vi "2D array remove NaN.vi"(1 "Data array":bool, 2 "2D array IN":dbl[][](array[numeric])=[[1.0, nan, 3.0], [1.0, 3.0, 4.0], [4.0, 5.0, nan], [5.0, 7.0, 6.0], [0.0, 0.0, 7.0]], 3 "delete Nan":bool) -> (0 "2D array cleaned":dbl[][](array[numeric])=[[1.0, 3.0, 4.0], [5.0, 7.0, 6.0], [0.0, 0.0, 7.0]])   [LabVIEW 2021]
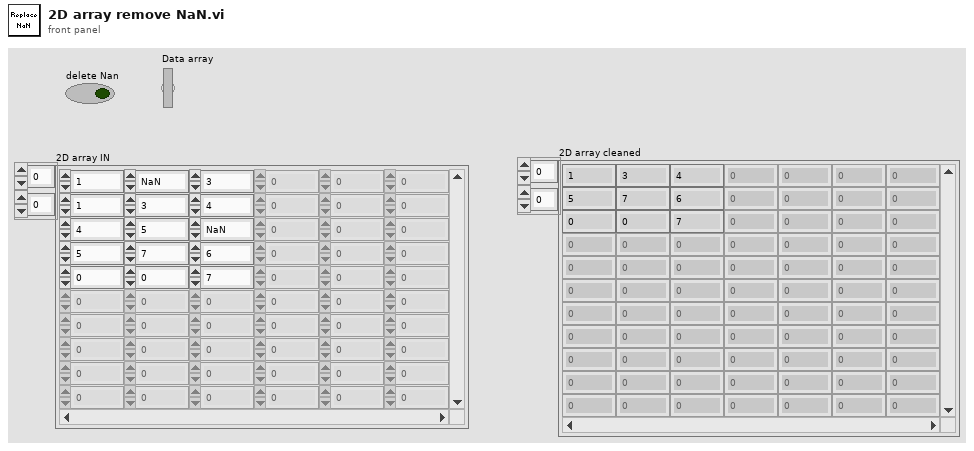
[diagram p1: front panel]
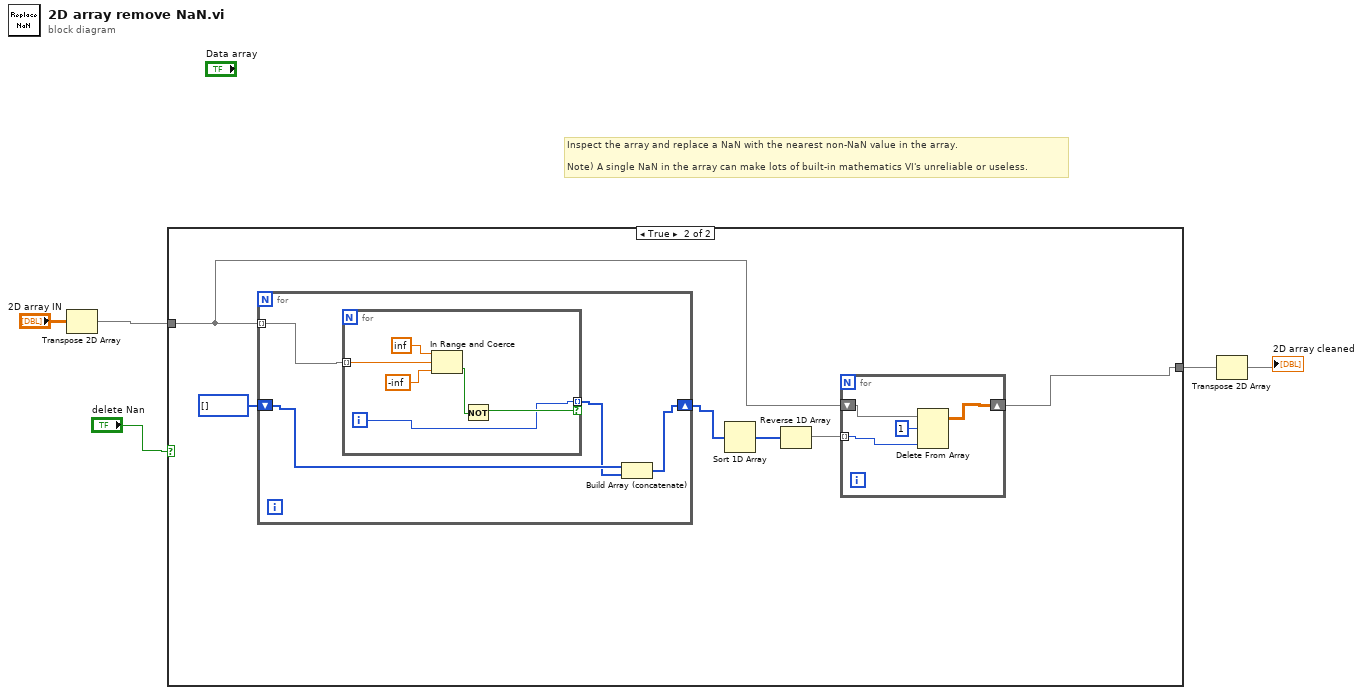
[diagram p0: block diagram]
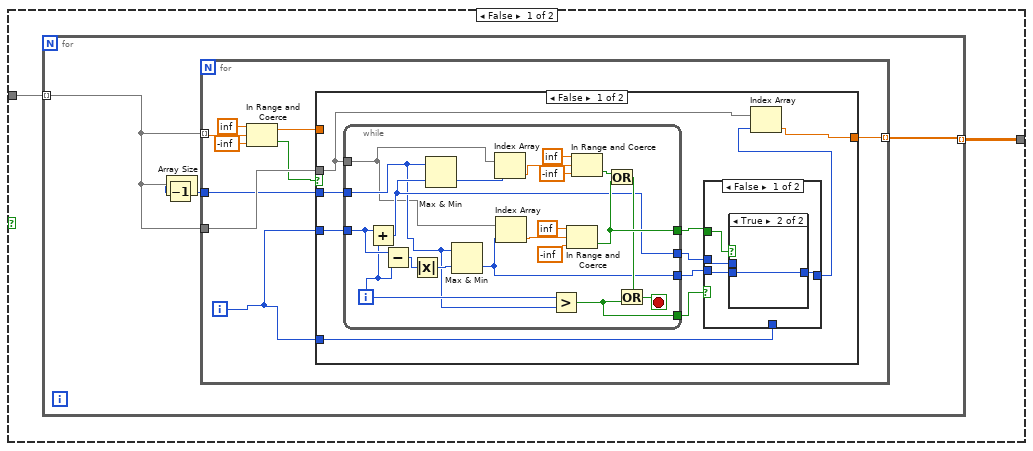
[diagram p2: hidden frame]
diagram:
  # "Inspect the array and replace a NaN with the nearest non-NaN value in the array.\n\nNote) A single NaN in the array can make lots of built-in mathematics VI's unreliable or useless."
  n1 = Transpose 2D Array(2D array="2D array IN") -> (transposed array=w3:dbl[][])
  n2 = case shown="True" "delete Nan" {
    tunnel: [w7 w59] -> w4
    tunnel: w3 -> [w6 w63]
    frame False {
      n3 = for {
        tunnel: w6 -> [w11] mode=indexing
        tunnel: [w10] -> w7 mode=indexing
        n4 = Array Size(array=w11) -> (size(s)=w9:i32)
        n5 = Decrement(x=w9) -> (x-1=w8:i32)
        n6 = for {
          tunnel: w11 -> [w18] mode=indexing
          tunnel: w11 -> [w17]
          tunnel: [w15] -> w10 mode=indexing
          tunnel: w8 -> [w12]
          i -> [w13]
          n7 = In Range and Coerce(upper limit=inf, x=w18, lower limit=-inf) -> (coerced(x)=w14:dbl, In Range?=w16:bool)
          n8 = case shown="False" w16 {
            tunnel: w17 -> [w29 _]
            tunnel: [w26 w58] -> w15
            tunnel: w14 -> [_ w58]
            tunnel: w13 -> [w30 _]
            tunnel: w13 -> [w23 _]
            tunnel: w12 -> [w21 _]
            frame False {
              n9 = while {
                tunnel: w29 -> [w38]
                tunnel: w30 -> [w54]
                tunnel: [w49] -> w22
                tunnel: [w40] -> w27
                tunnel: [w44] -> w25
                tunnel: [w45] -> w24
                tunnel: w21 -> [w39]
                i -> [w48]
                stop <- w46 stop-if-true
                n10 = Add(x=w54, y=w48) -> (x+y=w44:i32)
                n11 = Subtract(x=w54, y=w48) -> (x-y=w43:i32)
                n12 = Absolute Value(x=w43) -> (abs(x)=w41:i32)
                n13 = Max & Min(x=w39, y=w44) -> (min(x,y)=w42:i32)  [unwired: 1 out]
                n14 = Max & Min(x=w39, y=w41) -> (min(x,y)=w40:i32)  [unwired: 1 out]
                n15 = Index Array(array=w38, index=w42) -> (element=w55:dbl)
                n16 = Index Array(array=w38, index=w40) -> (element=w51:dbl)
                n17 = Greater?(x=w48, y=w39) -> (0:w45:bool)
                n18 = In Range and Coerce(upper limit=inf, x=w51, lower limit=-inf) -> (In Range?=w49:bool)  [unwired: 1 out]
                n19 = In Range and Coerce(upper limit=inf, x=w55, lower limit=-inf) -> (In Range?=w50:bool)  [unwired: 1 out]
                n20 = Or(x=w50, y=w49) -> (x .or. y?=w47:bool)
                n21 = Or(x=w47, y=w45) -> (x .or. y?=w46:bool)
              }
              n22 = case shown="False" w24 {
                tunnel: [w34 w37] -> w28
                tunnel: w27 -> [w33 _]
                tunnel: w25 -> [w32 _]
                tunnel: w23 -> [_ w37]
                tunnel: w22 -> [w31 _]
                frame False {
                  n23 = case shown="True" w31 {
                    tunnel: [w35 w36] -> w34
                    tunnel: w33 -> [_ w36]
                    tunnel: w32 -> [w35 _]
                    frame False {
                    }
                    frame True {
                    }
                  }
                }
                frame True {
                }
              }
              n24 = Index Array(array=w29, index=w28) -> (element=w26:dbl)
            }
            frame True {
            }
          }
        }
      }
    }
    frame True {
      n25 = for {
        tunnel: w63 -> [w72] mode=indexing
        shift-right: [w69] -> w62
        shift-left: i32[] [] -> [w71]
        n26 = for {
          tunnel: w72 -> [w76] mode=indexing
          tunnel: [w73] -> w70 mode=indexing if=w74
          i -> [w73]
          n27 = In Range and Coerce(upper limit=inf, x=w76, lower limit=-inf) -> (In Range?=w75:bool)  [unwired: 1 out]
          n28 = Not(x=w75) -> (.not. x?=w74:bool)
        }
        n29 = Build Array (concatenate)(w71, w70) -> (w69:i32[])
      }
      n30 = Sort 1D Array(array=w62) -> (sorted array=w61:i32[])
      n31 = Reverse 1D Array(array=w61) -> (reversed array=w60:i32[])
      n32 = for {
        shift-right: [w67] -> w59
        shift-left: w63 -> [w68]
        tunnel: w60 -> [w65] mode=indexing
        n33 = Delete From Array(array=w68, length=1, index (col)=w65) -> (array with subset deleted=w67:dbl[][])  [unwired: 1 in, 1 out]
      }
    }
  }
  n34 = Transpose 2D Array(2D array=w4) -> (transposed array=→"2D array cleaned":dbl[][])
